vi "CreatePath&FileName_noParamsinFileName.vi"(0 "FileName":string, 4 "Measurement type":T1(ring)) -> (1 "MeasurementGroupName":string, 2 "DatasetName":string, 3 "File path":path=path "Cluster Attributes.hdf5")   [LabVIEW 2019]
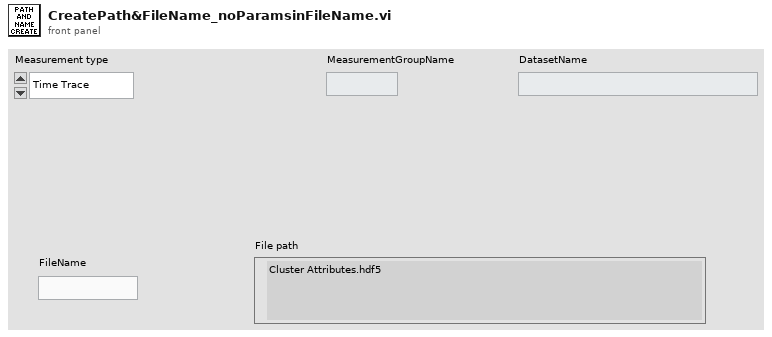
[diagram p1: front panel]
types:
  T1 = enum16{"Time Trace", "Contrast", "XY Intensity Map", "Polarisation", "Spectrum", "Michelson"}
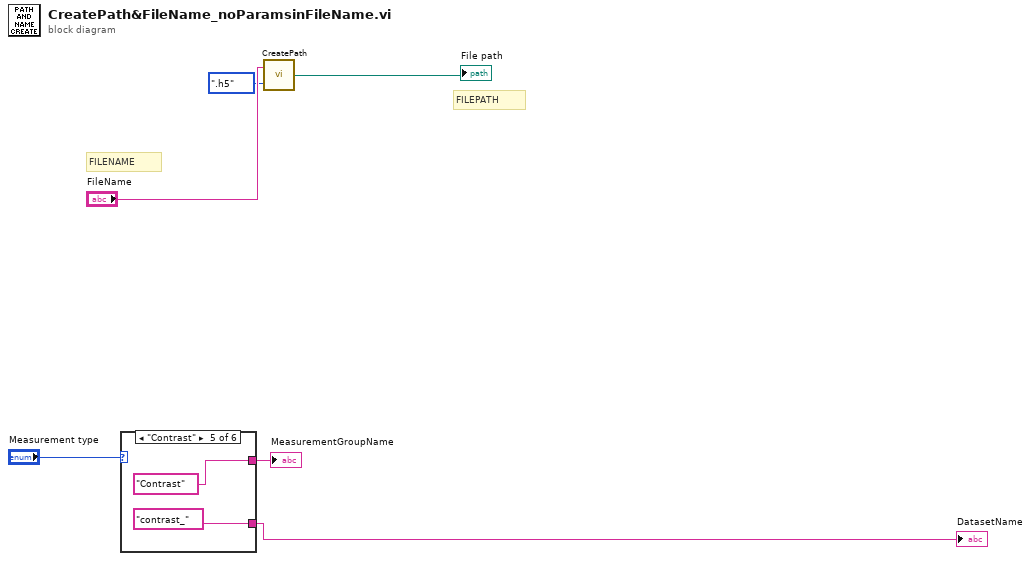
[diagram p0: block diagram]
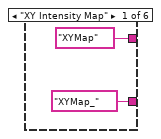
[diagram p2: hidden frame]
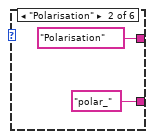
[diagram p3: hidden frame]
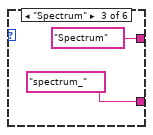
[diagram p4: hidden frame]
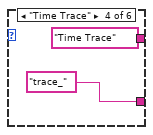
[diagram p5: hidden frame]
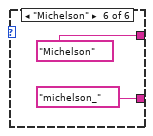
[diagram p6: hidden frame]
diagram:
  # "FILEPATH"
  # "FILENAME"
  n1 = case shown="\"Contrast\"" "Measurement type" {
    tunnel: ["XYMap" "Polarisation" "Spectrum" "Time Trace" "Contrast" "Michelson"] -> w5
    tunnel: ["XYMap_" "polar_" "spectrum_" "trace_" "contrast_" "michelson_"] -> w1
    frame "XY Intensity Map" {
    }
    frame "Polarisation" {
    }
    frame "Spectrum" {
    }
    frame "Time Trace" {
    }
    frame "Contrast" {
    }
    frame "Michelson" {
    }
  }
  "MeasurementGroupName" <- w5
  "DatasetName" <- w1
  n2 = call "CreatePath.vi"("filetype"=enum16{".h5", ".txt"}.".h5", "FileName"="FileName") -> ("File path"=→"File path":path)
